vi "Angle overlay.vi"(8 "error in (no error)":errorcluster, 10 "Overlay details in":T2={"Text factor"=0, "Xoffset"=0, "Arc size"=0.0, "Result"=0.0, "Line width"=0, "Measurment Name"="", "Angle"={"Point 1"={"X"=0.0, "Y"=0.0}, "Point 2"={"X"=0.0, "Y"=0.0}, "vertex"={"X"=0.0, "Y"=0.0}, "Point 1a"={"X"=0.0, "Y"=0.0}, "Point 2a"={"X"=0.0, "Y"=0.0}, "line1Point1"={"X"=0.0, "Y"=0.0}, "line1Point2"={"X"=0.0, "Y"=0.0}, "line2Point1"={"X"=0.0, "Y"=0.0}, "line2Point2"={"X"=0.0, "Y"=0.0}, "Angle type"="theta"}, "Maintain Width?"=FALSE, "Size factor"=0, "Colour"=0, "Mouse release point"={"X"=0.0, "Y"=0.0}, "Small FOV?"=FALSE, "Fixed FOV parameters"={"Inspection mode"=FALSE, "Overlay coordinates"=[], "Config coordinates"=[]}}, 11 "Image in":T1) -> (0 "error out":errorcluster, 1 "Overlay Coordinates out":cluster{"X":sgl, "Y":sgl}[](array[cluster]), 2 "Text origin":cluster{"X":sgl, "Y":sgl}, 3 "Image out":T1)   [LabVIEW 2019]
uses:
  <vilib>/vision/Image Controls.llb/IMAQ Image.ctl
  Controls/Angle details.ctl
  <vilib>/vision/NI_Vision_Development_Module.lvlib
panel:
  out "Error out":errorcluster
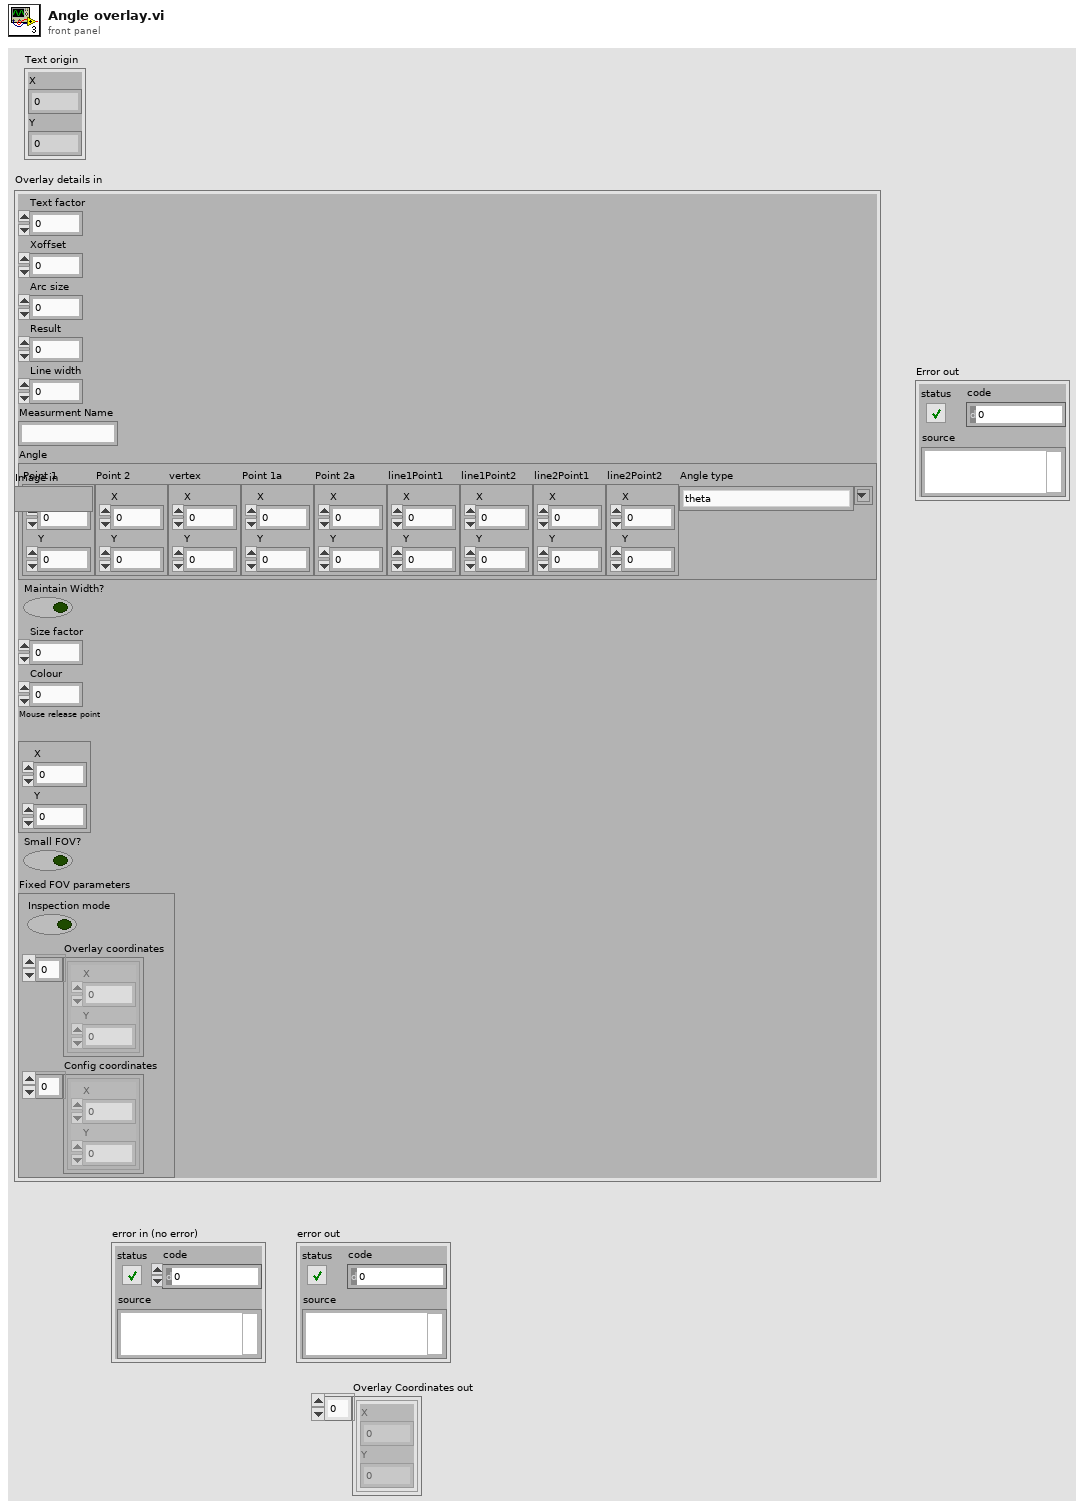
[diagram p1: front panel]
types:
  T1 = typedef "IMAQ Image.ctl" = refnum<image>
  T2 = typedef "Angle details.ctl" = cluster{"Text factor":u8, "Xoffset":i32, "Arc size":dbl, "Result":sgl, "Line width":i32, "Measurment Name":string, "Angle":cluster{"Point 1":cluster{"X":sgl, "Y":sgl}, "Point 2":cluster{"X":sgl, "Y":sgl}, "vertex":cluster{"X":sgl, "Y":sgl}, "Point 1a":cluster{"X":sgl, "Y":sgl}, "Point 2a":cluster{"X":sgl, "Y":sgl}, "line1Point1":cluster{"X":sgl, "Y":sgl}, "line1Point2":cluster{"X":sgl, "Y":sgl}, "line2Point1":cluster{"X":sgl, "Y":sgl}, "line2Point2":cluster{"X":sgl, "Y":sgl}, "Angle type":string}, "Maintain Width?":bool, "Size factor":u32, "Colour":u32, "Mouse release point":cluster{"X":sgl, "Y":sgl}, "Small FOV?":bool, "Fixed FOV parameters":cluster{"Inspection mode":bool, "Overlay coordinates":cluster{"X":sgl, "Y":sgl}[], "Config coordinates":cluster{"X":sgl, "Y":sgl}[]}}
  T3 = cluster{"Point 1":cluster{"X":sgl, "Y":sgl}, "Point 2":cluster{"X":sgl, "Y":sgl}}
  T4 = cluster{"Desired Font (Application)":enum16{"User-specified Font", "Application Font", "System Font", "Dialog Font"}, "[User-specified Font]":cluster{"Font Name":string, "Size":i16, "Strikeout?":bool, "Italic?":bool, "Underline?":bool, "Outline?":bool, "Shadow?":bool, "Bold?":bool, "Rotation Angle":dbl}, "Horizontal Alignment":i16, "Vertical Alignment":i16}
  T5 = cluster{"Point 1":cluster{"X":sgl, "Y":sgl}, "Point 2":cluster{"X":sgl, "Y":sgl}, "vertex":cluster{"X":sgl, "Y":sgl}, "Point 1a":cluster{"X":sgl, "Y":sgl}, "Point 2a":cluster{"X":sgl, "Y":sgl}, "line1Point1":cluster{"X":sgl, "Y":sgl}, "line1Point2":cluster{"X":sgl, "Y":sgl}, "line2Point1":cluster{"X":sgl, "Y":sgl}, "line2Point2":cluster{"X":sgl, "Y":sgl}, "Angle type":string}
  T6 = cluster{"Inspection mode":bool, "Overlay coordinates":cluster{"X":sgl, "Y":sgl}[], "Config coordinates":cluster{"X":sgl, "Y":sgl}[]}
  T7 = typedef "IMAQ Line" = cluster{"Start X":i32, "Start Y":i32, "End X":i32, "End Y":i32}
  T8 = cluster{"Left":i32, "Top":i32, "Right":i32, "Bottom":i32}
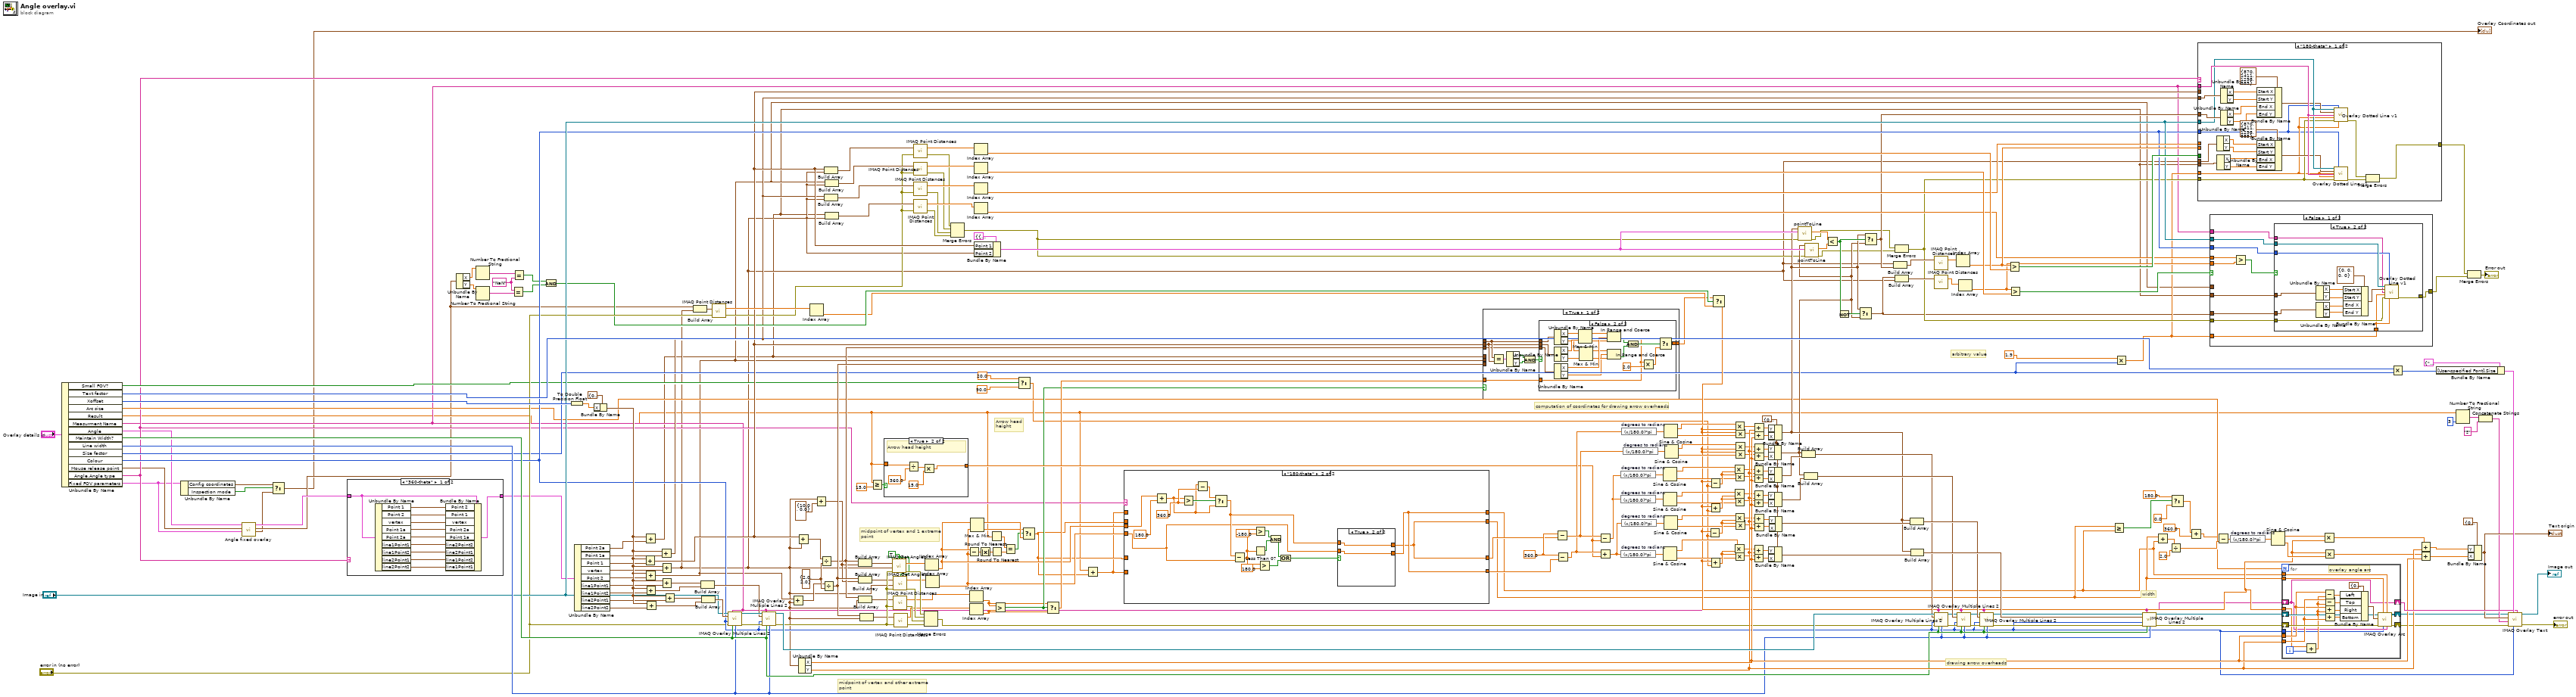
[diagram p0: block diagram]
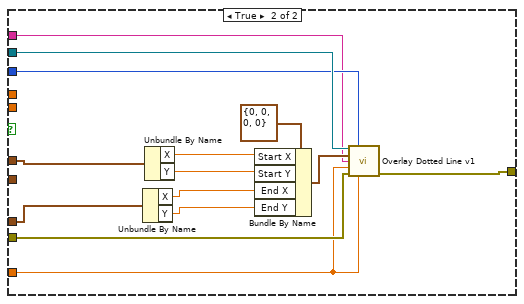
[diagram p3: hidden frame]
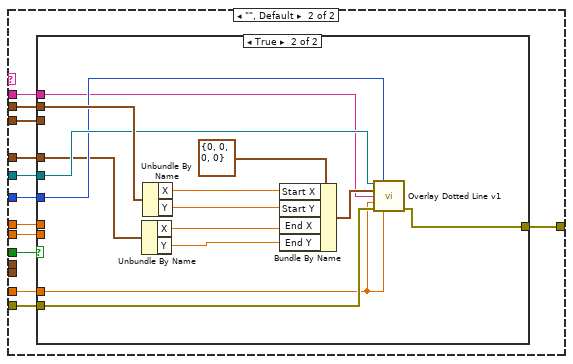
[diagram p4: hidden frame]
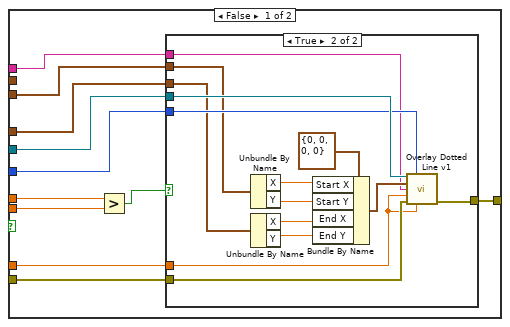
[diagram p5: hidden frame]
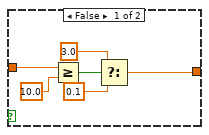
[diagram p10: hidden frame]
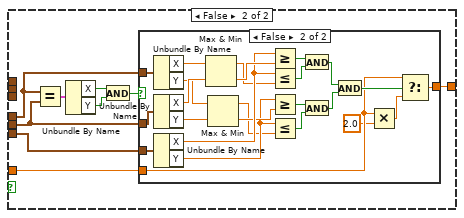
[diagram p12: hidden frame]
diagram:
  w48 = "NaN" ("x")
  w216 = 360.0 ("x")
  w198 = cluster{"X":sgl, "Y":sgl} {"X"=0.0, "Y"=0.0} ("y")
  w136 = cluster{"X":sgl, "Y":sgl} {"X"=2.0, "Y"=2.0} ("y")
  w110 = TRUE ("Use Vertex (No)")
  # "arbitrary value"
  # "Arrow head\nheight"
  # "midpoint of vertex and other extreme\npoint"
  # "midpoint of vertex and 1 extreme\npoint"
  # "drawing arrow overheads"
  # "computation of coordinates for drawing arrow overheads"
  # "width"
  n1 = Unbundle By Name("Overlay details in") -> ("Small FOV?"=w37:bool, "Text factor"=w104:u8, "Xoffset"=w103:i32, "Arc size"=w38:dbl, "Result"=w18:sgl, "Measurment Name"=w22:string, "Angle"=w9:T5, "Maintain Width?"=w102:bool, "Line width"=w101:i32, "Size factor"=w41:u32, "Colour"=w79:u32, "Mouse release point"=w7:cluster{"X":sgl, "Y":sgl}, "Angle.Angle type"=w23:string, "Fixed FOV parameters"=w5:T6)
  n2 = Unbundle By Name(w5) -> ("Config coordinates"=w3:cluster{"X":sgl, "Y":sgl}[], "Inspection mode"=w2:bool)
  n3 = call "Angle fixed overlay.vi"("Fixed FOV parameters"=w5, "Mouse release point"=w7, "Angle"=w9) -> ("Overlay Coordinates"=w4:cluster{"X":sgl, "Y":sgl}[], "Mouse release point out"=w6:cluster{"X":sgl, "Y":sgl}, "Angle parameters out"=w8:T5)  [unwired: 6 in]
  n4 = Select(t=w3, s=w2, f=w4) -> (s? t:f=→"Overlay Coordinates out":cluster{"X":sgl, "Y":sgl}[])
  n5 = case shown="\"360-theta\"" w23 {
    tunnel: w8 -> [w266 w267]
    tunnel: [w265 w267] -> w31
    frame "360-theta" {
      n6 = Unbundle By Name(w266) -> ("Point 1"=w264:cluster{"X":sgl, "Y":sgl}, "Point 2"=w263:cluster{"X":sgl, "Y":sgl}, "vertex"=w262:cluster{"X":sgl, "Y":sgl}, "Point 1a"=w261:cluster{"X":sgl, "Y":sgl}, "Point 2a"=w260:cluster{"X":sgl, "Y":sgl}, "line1Point1"=w259:cluster{"X":sgl, "Y":sgl}, "line1Point2"=w258:cluster{"X":sgl, "Y":sgl}, "line2Point1"=w257:cluster{"X":sgl, "Y":sgl}, "line2Point2"=w256:cluster{"X":sgl, "Y":sgl})
      n7 = Bundle By Name(cluster=w266, "Point 2"=w264, "Point 1"=w263, "vertex"=w262, "Point 2a"=w261, "Point 1a"=w260, "line2Point2"=w259, "line2Point1"=w258, "line1Point2"=w257, "line1Point1"=w256) -> (w265:T5)
    }
    frame "theta", Default {
    }
  }
  n8 = Unbundle By Name(w6) -> ("X"=w52:sgl, "Y"=w51:sgl)
  n9 = Number To Fractional String(number=w52) -> (F-format string=w50:string)  [unwired: 3 in]
  n10 = Number To Fractional String(number=w51) -> (F-format string=w49:string)  [unwired: 3 in]
  n11 = Equal?(x=w48, y=w49) -> (x = y?=w46:bool)
  n12 = Equal?(x=w50, y=w48) -> (x = y?=w47:bool)
  n13 = And(x=w47, y=w46) -> (x .and. y?=w45:bool)
  n14 = To Double Precision Float(number=w103) -> (double precision float=w234:dbl)
  n15 = Unbundle By Name(w31) -> ("Point 2a"=w235:cluster{"X":sgl, "Y":sgl}, "Point 1a"=w236:cluster{"X":sgl, "Y":sgl}, "Point 1"=w237:cluster{"X":sgl, "Y":sgl}, "vertex"=w33:cluster{"X":sgl, "Y":sgl}, "Point 2"=w238:cluster{"X":sgl, "Y":sgl}, "line1Point1"=w239:cluster{"X":sgl, "Y":sgl}, "line1Point2"=w241:cluster{"X":sgl, "Y":sgl}, "line2Point1"=w243:cluster{"X":sgl, "Y":sgl}, "line2Point2"=w246:cluster{"X":sgl, "Y":sgl})
  n16 = Bundle By Name(cluster=cluster{"X":sgl, "Y":sgl} {"X"=0.0, "Y"=0.0} ("Angle.Point 2a"), "X"=w234) -> (w245:cluster{"X":sgl, "Y":sgl})
  n17 = Add(x=w245, y=w237) -> (x+y=w75:cluster{"X":sgl, "Y":sgl})
  n18 = Add(x=w245, y=w235) -> (x+y=w19:cluster{"X":sgl, "Y":sgl})
  n19 = Add(x=w245, y=w238) -> (x+y=w21:cluster{"X":sgl, "Y":sgl})
  n20 = Add(x=w245, y=w241) -> (x+y=w242:cluster{"X":sgl, "Y":sgl})
  n21 = Add(x=w245, y=w246) -> (x+y=w247:cluster{"X":sgl, "Y":sgl})
  n22 = Add(x=w245, y=w236) -> (x+y=w24:cluster{"X":sgl, "Y":sgl})
  n23 = Add(x=w245, y=w33) -> (x+y=w20:cluster{"X":sgl, "Y":sgl})
  n24 = Add(x=w245, y=w239) -> (x+y=w240:cluster{"X":sgl, "Y":sgl})
  n25 = Add(x=w245, y=w243) -> (x+y=w244:cluster{"X":sgl, "Y":sgl})
  n26 = Build Array(w6, w20) -> (w78:cluster{"X":sgl, "Y":sgl}[])
  n27 = Build Array(w240, w242) -> (w232:cluster{"X":sgl, "Y":sgl}[])
  n28 = Build Array(w244, w247) -> (w248:cluster{"X":sgl, "Y":sgl}[])
  n29 = call "IMAQ Point Distances"("Points"=w78, "error in (no error)"="error in (no error)") -> ("Distances"=w77:sgl[], "error out"=w58:errorcluster)  [unwired: 3 in]
  n30 = call "IMAQ Overlay Multiple Lines 2"("Image"="Image in", "Group"=w22, "Line End Points"=w248, "Color"=w79, "error in (no error)"="error in (no error)", "Maintain Width?"=w102, "Width"=w101) -> ("Image Out"=w252:T1, "error out"=w251:errorcluster)  [unwired: 7 in]
  n31 = call "IMAQ Overlay Multiple Lines 2"("Image"=w252, "Group"=w22, "Line End Points"=w232, "Color"=w79, "error in (no error)"=w251, "Maintain Width?"=w102, "Width"=w101) -> ("Image Out"=w231:T1, "error out"=w230:errorcluster)  [unwired: 7 in]
  n32 = Add(x=w21, y=w20) -> (x+y=w135:cluster{"X":sgl, "Y":sgl})
  n33 = Add(x=w75, y=w20) -> (x+y=w219:cluster{"X":sgl, "Y":sgl})
  n34 = Unbundle By Name(w20) -> ("X"=w200:sgl, "Y"=w199:sgl)
  n35 = Index Array(array=w77) -> (element=w43:sgl)  [unwired: 1 in]
  n36 = Add(x=w20, y=cluster{"X":sgl, "Y":sgl} {"X"=10.0, "Y"=0.0}) -> (x+y=w109:cluster{"X":sgl, "Y":sgl})
  n37 = Divide(x=w219, y=w136) -> (x/y=w154:cluster{"X":sgl, "Y":sgl})
  n38 = Divide(x=w135, y=w136) -> (x/y=w155:cluster{"X":sgl, "Y":sgl})
  n39 = Build Array(w75, w20) -> (w100:cluster{"X":sgl, "Y":sgl}[])
  n40 = Build Array(w24, w20) -> (w98:cluster{"X":sgl, "Y":sgl}[])
  n41 = Build Array(w21, w20) -> (w99:cluster{"X":sgl, "Y":sgl}[])
  n42 = Build Array(w19, w20) -> (w97:cluster{"X":sgl, "Y":sgl}[])
  n43 = Build Array(w154, w109) -> (w106:cluster{"X":sgl, "Y":sgl}[])
  n44 = Build Array(w155, w109) -> (w107:cluster{"X":sgl, "Y":sgl}[])
  n45 = Build Array(w154, w20) -> (w113:cluster{"X":sgl, "Y":sgl}[])
  n46 = Build Array(w155, w20) -> (w114:cluster{"X":sgl, "Y":sgl}[])
  n47 = Greater Or Equal?(x=w18, y=sgl 15.0) -> (x >= y?=w176:bool)
  n48 = case shown="True" w176 {
    tunnel: w18 -> [w273 w278]
    tunnel: [w268 w274] -> w177
    frame False {
      n49 = Greater Or Equal?(x=w273, y=sgl 10.0) -> (x >= y?=w271:bool)
      n50 = Select(t=3.0, s=w271, f=0.1) -> (s? t:f=w268:dbl)
    }
    frame True {
      # "Arrow head height"
      n51 = Divide(x=w278, y=sgl 360.0) -> (x/y=w276:sgl)
      n52 = Multiply(x=w276, y=sgl 15.0) -> (x*y=w274:sgl)
    }
  }
  n53 = call "IMAQ Get Angles"("error in (no error)"=w230, "Vertex"=w20, "Points"=w106, "Use Vertex (No)"=w110) -> ("error out"=w141:errorcluster, "Angles (deg)"=w111:sgl[])  [unwired: 1 in, 1 out]
  n54 = call "IMAQ Get Angles"("error in (no error)"=w230, "Vertex"=w20, "Points"=w107, "Use Vertex (No)"=w110) -> ("error out"=w140:errorcluster, "Angles (deg)"=w112:sgl[])  [unwired: 1 in, 1 out]
  n55 = call "IMAQ Point Distances"("Points"=w113, "error in (no error)"=w230) -> ("Distances"=w115:sgl[], "error out"=w139:errorcluster)  [unwired: 3 in]
  n56 = call "IMAQ Point Distances"("Points"=w114, "error in (no error)"=w230) -> ("Distances"=w116:sgl[], "error out"=w138:errorcluster)  [unwired: 3 in]
  n57 = call "IMAQ Point Distances"("Points"=w100, "error in (no error)"=w58) -> ("Distances"=w94:sgl[], "error out"=w54:errorcluster)  [unwired: 3 in]
  n58 = call "IMAQ Point Distances"("Points"=w98, "error in (no error)"=w58) -> ("Distances"=w92:sgl[], "error out"=w56:errorcluster)  [unwired: 3 in]
  n59 = call "IMAQ Point Distances"("Points"=w99, "error in (no error)"=w58) -> ("Distances"=w93:sgl[], "error out"=w55:errorcluster)  [unwired: 3 in]
  n60 = call "IMAQ Point Distances"("Points"=w97, "error in (no error)"=w58) -> ("Distances"=w91:sgl[], "error out"=w57:errorcluster)  [unwired: 3 in]
  n61 = Merge Errors(w141, w140, w139, w138) -> (w66:errorcluster)
  n62 = Index Array(array=w111) -> (element=w30:sgl)  [unwired: 1 in]
  n63 = Index Array(array=w112) -> (element=w29:sgl)  [unwired: 1 in]
  n64 = Merge Errors(w54, w55, w56, w57) -> (w53:errorcluster)
  n65 = Subtract(x=w30, y=w29) -> (x-y=w223:sgl)
  n66 = Index Array(array=w115) -> (element=w117:sgl)  [unwired: 1 in]
  n67 = Index Array(array=w116) -> (element=w118:sgl)  [unwired: 1 in]
  n68 = Max & Min(x=w30, y=w29) -> (max(x,y)=w226:sgl, min(x,y)=w225:sgl)
  n69 = Index Array(array=w94) -> (element=w89:sgl)  [unwired: 1 in]
  n70 = Index Array(array=w93) -> (element=w87:sgl)  [unwired: 1 in]
  n71 = Index Array(array=w92) -> (element=w84:sgl)  [unwired: 1 in]
  n72 = Index Array(array=w91) -> (element=w82:sgl)  [unwired: 1 in]
  n73 = Bundle By Name(cluster=T3 {"Point 1"={"X"=0.0, "Y"=0.0}, "Point 2"={"X"=0.0, "Y"=0.0}} ("Line"), "Point 1"=w75, "Point 2"=w20) -> (w74:T3)
  n74 = Absolute Value(x=w223) -> (abs(x)=w228:sgl)
  n75 = Round To Nearest(number=w18) -> (nearest integer value=w229:sgl)
  n76 = Round To Nearest(number=w228) -> (nearest integer value=w227:sgl)
  n77 = Greater?(x=w117, y=w118) -> (0:w153:bool)
  n78 = Equal?(x=w229, y=w227) -> (x = y?=w224:bool)
  n79 = Select(t=sgl 20.0 ("y"), s=w37, f=sgl 90.0 ("y")) -> (s? t:f=w34:sgl)
  n80 = Select(t=w225, s=w224, f=w226) -> (s? t:f=w28:sgl)
  n81 = Select(t=w117, s=w153, f=w118) -> (s? t:f=w156:sgl)
  n82 = Add(x=w18, y=w28) -> (x+y=w26:sgl)
  n83 = case shown="\"180-theta\"" w23 {
    tunnel: w28 -> [w281 _]
    tunnel: w26 -> [w282 _]
    tunnel: w30 -> [_ w295]
    tunnel: w29 -> [_ w290]
    tunnel: [w282 w289] -> w11
    tunnel: [w281 w288] -> w12
    tunnel: w28 -> [w280 _]
    tunnel: [w280 w288] -> w27
    tunnel: [w279 w289] -> w25
    tunnel: w26 -> [w279 _]
    frame "", Default {
    }
    frame "180-theta" {
      w297 = sgl 360.0 ("y")
      n84 = Add(x=w295, y=sgl 180.0) -> (x+y=w296:sgl)
      n85 = Greater?(x=w296, y=w297) -> (0:w299:bool)
      n86 = Subtract(x=w296, y=w297) -> (x-y=w298:sgl)
      n87 = Select(t=w298, s=w299, f=w296) -> (s? t:f=w291:sgl)
      n88 = Subtract(x=w291, y=w290) -> (x-y=w287:sgl)
      n89 = Greater?(x=w287, y=sgl -180.0) -> (0:w285:bool)
      n90 = Less Than 0?(x=w287) -> (x < 0?=w284:bool)
      n91 = Greater?(x=w287, y=sgl 180.0) -> (0:w293:bool)
      n92 = And(x=w285, y=w284) -> (x .and. y?=w283:bool)
      n93 = Or(x=w283, y=w293) -> (x .or. y?=w292:bool)
      n94 = case shown="True" w292 {
        tunnel: w291 -> [w302 w303]
        tunnel: w290 -> [w301 w304]
        tunnel: [w302 w304] -> w289
        tunnel: [w301 w303] -> w288
        frame False {
        }
        frame True {
        }
      }
    }
  }
  n95 = case shown="True" w153 {
    tunnel: w75 -> [w310 _]
    tunnel: w24 -> [w311 _]
    tunnel: w21 -> [_ w339]
    tunnel: w19 -> [_ w340]
    tunnel: w154 -> [w305 _]
    tunnel: w155 -> [_ w341]
    tunnel: w156 -> [w312 w343]
    tunnel: [w313 w342] -> w42
    frame True {
      n96 = Equal?(x=w311, y=w310) -> (x = y?=w309:cluster{"X":bool, "Y":bool})
      n97 = Unbundle By Name(w309) -> ("X"=w308:bool, "Y"=w307:bool)
      n98 = And(x=w308, y=w307) -> (x .and. y?=w306:bool)
      n99 = case shown="False" w306 {
        tunnel: w305 -> [_ w334]
        tunnel: [w314 w326] -> w313
        tunnel: w312 -> [w314 w325]
        tunnel: w311 -> [_ w324]
        tunnel: w310 -> [_ w323]
        frame True {
        }
        frame False {
          n100 = Unbundle By Name(w324) -> ("X"=w333:sgl, "Y"=w331:sgl)
          n101 = Unbundle By Name(w323) -> ("X"=w332:sgl, "Y"=w330:sgl)
          n102 = Unbundle By Name(w334) -> ("X"=w321:sgl, "Y"=w316:sgl)
          n103 = Max & Min(x=w333, y=w332) -> (max(x,y)=w322:sgl, min(x,y)=w320:sgl)
          n104 = Max & Min(x=w331, y=w330) -> (max(x,y)=w318:sgl, min(x,y)=w317:sgl)
          n105 = In Range and Coerce(upper limit=w322, x=w321, lower limit=w320) -> (In Range?=w319:bool)  [unwired: 1 out]
          n106 = In Range and Coerce(upper limit=w318, x=w316, lower limit=w317) -> (In Range?=w315:bool)  [unwired: 1 out]
          n107 = And(x=w319, y=w315) -> (x .and. y?=w329:bool)
          n108 = Multiply(x=w325, y=sgl 2.0) -> (x*y=w328:sgl)
          n109 = Select(t=w325, s=w329, f=w328) -> (s? t:f=w326:sgl)
        }
      }
    }
    frame False {
      n110 = Equal?(x=w340, y=w339) -> (x = y?=w338:cluster{"X":bool, "Y":bool})
      n111 = Unbundle By Name(w338) -> ("X"=w337:bool, "Y"=w336:bool)
      n112 = And(x=w337, y=w336) -> (x .and. y?=w335:bool)
      n113 = case shown="False" w335 {
        tunnel: w343 -> [w344 w350]
        tunnel: [w344 w348] -> w342
        tunnel: w341 -> [_ w347]
        tunnel: w340 -> [_ w346]
        tunnel: w339 -> [_ w345]
        frame True {
        }
        frame False {
          n114 = Unbundle By Name(w346) -> ("X"=w368:sgl, "Y"=w366:sgl)
          n115 = Unbundle By Name(w345) -> ("X"=w367:sgl, "Y"=w365:sgl)
          n116 = Unbundle By Name(w347) -> ("X"=w363:sgl, "Y"=w356:sgl)
          n117 = Max & Min(x=w368, y=w367) -> (max(x,y)=w362:sgl, min(x,y)=w364:sgl)
          n118 = Max & Min(x=w366, y=w365) -> (max(x,y)=w355:sgl, min(x,y)=w357:sgl)
          n119 = Greater Or Equal?(x=w363, y=w364) -> (x >= y?=w361:bool)
          n120 = Less Or Equal?(x=w363, y=w362) -> (x <= y?=w360:bool)
          n121 = Greater Or Equal?(x=w356, y=w357) -> (x >= y?=w358:bool)
          n122 = Less Or Equal?(x=w356, y=w355) -> (x <= y?=w359:bool)
          n123 = And(x=w361, y=w360) -> (x .and. y?=w353:bool)
          n124 = And(x=w358, y=w359) -> (x .and. y?=w354:bool)
          n125 = And(x=w353, y=w354) -> (x .and. y?=w352:bool)
          n126 = Multiply(x=w350, y=sgl 2.0) -> (x*y=w351:sgl)
          n127 = Select(t=w350, s=w352, f=w351) -> (s? t:f=w348:sgl)
        }
      }
    }
  }
  n128 = Subtract(x=w216, y=w27) -> (x-y=w218:dbl)
  n129 = Subtract(x=w216, y=w25) -> (x-y=w217:dbl)
  n130 = Subtract(x=w218, y=w177) -> (x-y=w249:dbl)
  n131 = Add(x=w217, y=w177) -> (x+y=w215:dbl)
  n132 = expression code="(x/180.0)*pi" "degrees to radians"(w249) -> (w157:dbl)
  n133 = expression code="(x/180.0)*pi" "degrees to radians"(w249) -> (w181:dbl)
  n134 = expression code="(x/180.0)*pi" "degrees to radians"(w215) -> (w190:dbl)
  n135 = expression code="(x/180.0)*pi" "degrees to radians"(w217) -> (w143:dbl)
  n136 = expression code="(x/180.0)*pi" "degrees to radians"(w215) -> (w162:dbl)
  n137 = expression code="(x/180.0)*pi" "degrees to radians"(w218) -> (w144:dbl)
  n138 = Sine & Cosine(0:w157) -> (1:w158:dbl, 2:w159:dbl)
  n139 = Sine & Cosine(0:w181) -> (1:w182:dbl, 2:w183:dbl)
  n140 = Sine & Cosine(0:w190) -> (1:w191:dbl, 2:w192:dbl)
  n141 = Sine & Cosine(0:w143) -> (1:w145:dbl, 2:w146:dbl)
  n142 = Sine & Cosine(0:w162) -> (1:w163:dbl, 2:w164:dbl)
  n143 = Sine & Cosine(0:w144) -> (1:w147:dbl, 2:w148:dbl)
  n144 = Select(t=w42, s=w45, f=w43) -> (s? t:f=w44:sgl)
  n145 = Subtract(x=w44, y=w34) -> (x-y=w189:sgl)
  n146 = Subtract(x=w44, y=w34) -> (x-y=w180:sgl)
  n147 = Add(x=w44, y=w34) -> (x+y=w188:sgl)
  n148 = Add(x=w44, y=w34) -> (x+y=w197:sgl)
  n149 = Multiply(x=w158, y=w180) -> (x*y=w160:dbl)
  n150 = Multiply(x=w182, y=w188) -> (x*y=w184:dbl)
  n151 = Multiply(x=w191, y=w197) -> (x*y=w193:dbl)
  n152 = Multiply(x=w145, y=w44) -> (x*y=w149:dbl)
  n153 = Multiply(x=w180, y=w159) -> (x*y=w161:dbl)
  n154 = Multiply(x=w188, y=w183) -> (x*y=w185:dbl)
  n155 = Multiply(x=w163, y=w189) -> (x*y=w165:dbl)
  n156 = Multiply(x=w197, y=w192) -> (x*y=w194:dbl)
  n157 = Multiply(x=w44, y=w146) -> (x*y=w150:dbl)
  n158 = Multiply(x=w147, y=w44) -> (x*y=w151:dbl)
  n159 = Multiply(x=w44, y=w148) -> (x*y=w152:dbl)
  n160 = Multiply(x=w189, y=w164) -> (x*y=w166:dbl)
  n161 = Add(x=w160, y=w199) -> (x+y=w171:dbl)
  n162 = Add(x=w161, y=w200) -> (x+y=w172:dbl)
  n163 = Add(x=w184, y=w199) -> (x+y=w186:dbl)
  n164 = Add(x=w185, y=w200) -> (x+y=w187:dbl)
  n165 = Add(x=w193, y=w199) -> (x+y=w195:dbl)
  n166 = Add(x=w194, y=w200) -> (x+y=w196:dbl)
  n167 = Add(x=w149, y=w199) -> (x+y=w167:dbl)
  n168 = Add(x=w150, y=w200) -> (x+y=w168:dbl)
  n169 = Add(x=w151, y=w199) -> (x+y=w169:dbl)
  n170 = Add(x=w152, y=w200) -> (x+y=w170:dbl)
  n171 = Add(x=w165, y=w199) -> (x+y=w173:dbl)
  n172 = Add(x=w166, y=w200) -> (x+y=w174:dbl)
  n173 = Bundle By Name(cluster=w198, "Y"=w169, "X"=w170) -> (w68:cluster{"X":sgl, "Y":sgl})
  n174 = Bundle By Name(cluster=w198, "Y"=w167, "X"=w168) -> (w69:cluster{"X":sgl, "Y":sgl})
  n175 = Bundle By Name(cluster=w198, "Y"=w171, "X"=w172) -> (w201:cluster{"X":sgl, "Y":sgl})
  n176 = Bundle By Name(cluster=w198, "Y"=w186, "X"=w187) -> (w202:cluster{"X":sgl, "Y":sgl})
  n177 = Bundle By Name(cluster=w198, "Y"=w195, "X"=w196) -> (w204:cluster{"X":sgl, "Y":sgl})
  n178 = Bundle By Name(cluster=w198, "Y"=w173, "X"=w174) -> (w203:cluster{"X":sgl, "Y":sgl})
  n179 = call "pointToLine.vi"("error in (no error)"=w53, "Line"=w74, "Point"=w69) -> ("error out"=w64:errorcluster, "distance"=w73:dbl)  [unwired: 6 in, 1 out]
  n180 = Build Array(w68, w201) -> (w211:cluster{"X":sgl, "Y":sgl}[])
  n181 = Build Array(w68, w202) -> (w212:cluster{"X":sgl, "Y":sgl}[])
  n182 = call "pointToLine.vi"("error in (no error)"=w53, "Line"=w74, "Point"=w68) -> ("error out"=w65:errorcluster, "distance"=w72:dbl)  [unwired: 6 in, 1 out]
  n183 = Less?(x=w73, y=w72) -> (x < y?=w71:bool)
  n184 = Not(x=w71) -> (.not. x?=w70:bool)
  n185 = Select(t=w69, s=w70, f=w68) -> (s? t:f=w32:cluster{"X":sgl, "Y":sgl})
  n186 = Select(t=w69, s=w71, f=w68) -> (s? t:f=w67:cluster{"X":sgl, "Y":sgl})
  n187 = Build Array(w20, w67) -> (w96:cluster{"X":sgl, "Y":sgl}[])
  n188 = Build Array(w32, w20) -> (w95:cluster{"X":sgl, "Y":sgl}[])
  n189 = Merge Errors(w64, w65) -> (w63:errorcluster)
  n190 = Build Array(w69, w203) -> (w213:cluster{"X":sgl, "Y":sgl}[])
  n191 = Build Array(w69, w204) -> (w214:cluster{"X":sgl, "Y":sgl}[])
  n192 = call "IMAQ Point Distances"("Points"=w96) -> ("Distances"=w90:sgl[])  [unwired: 4 in, 1 out]
  n193 = call "IMAQ Overlay Multiple Lines 2"("Image"=w231, "Group"=w22, "Line End Points"=w211, "Color"=w79, "error in (no error)"=w66, "Maintain Width?"=w102, "Width"=w101) -> ("Image Out"=w179:T1, "error out"=w178:errorcluster)  [unwired: 7 in]
  n194 = call "IMAQ Point Distances"("Points"=w95) -> ("Distances"=w88:sgl[])  [unwired: 4 in, 1 out]
  n195 = Index Array(array=w90) -> (element=w83:sgl)  [unwired: 1 in]
  n196 = call "IMAQ Overlay Multiple Lines 2"("Image"=w179, "Group"=w22, "Line End Points"=w212, "Color"=w79, "error in (no error)"=w178, "Maintain Width?"=w102, "Width"=w101) -> ("Image Out"=w206:T1, "error out"=w205:errorcluster)  [unwired: 7 in]
  n197 = Index Array(array=w88) -> (element=w81:sgl)  [unwired: 1 in]
  n198 = call "IMAQ Overlay Multiple Lines 2"("Image"=w206, "Group"=w22, "Line End Points"=w213, "Color"=w79, "error in (no error)"=w205, "Maintain Width?"=w102, "Width"=w101) -> ("Image Out"=w209:T1, "error out"=w207:errorcluster)  [unwired: 7 in]
  n199 = Greater?(x=w83, y=w89) -> (0:w86:bool)
  n200 = Greater?(x=w81, y=w87) -> (0:w85:bool)
  n201 = Greater Or Equal?(x=w12, y=w11) -> (x >= y?=w10:bool)
  n202 = Multiply(x=1.9, y=w41) -> (x*y=w40:dbl)
  n203 = call "IMAQ Overlay Multiple Lines 2"("Image"=w209, "Group"=w22, "Line End Points"=w214, "Color"=w79, "error in (no error)"=w207, "Maintain Width?"=w102, "Width"=w101) -> ("Image Out"=w210:T1, "error out"=w208:errorcluster)  [unwired: 7 in]
  n204 = Add(x=w12, y=w11) -> (x+y=w124:sgl)
  n205 = Divide(x=w124, y=2.0) -> (x/y=w221:dbl)
  n206 = Select(t=180.0, s=w10, f=0.0) -> (s? t:f=w13:dbl)
  n207 = Add(x=w13, y=360.0 ("x")) -> (x+y=w17:dbl)
  n208 = case shown="\"180-theta\"" w23 {
    tunnel: w86 -> [_ w404]
    tunnel: w84 -> [_ w403]
    tunnel: w83 -> [_ w402]
    tunnel: "Image in" -> [w377 w401]
    tunnel: w79 -> [w369 w400]
    tunnel: w75 -> [_ w399]
    tunnel: w67 -> [w391 w398]
    tunnel: w63 -> [w374 w397]
    tunnel: [w371 w396] -> w61
    tunnel: w40 -> [w373 w395]
    tunnel: w22 -> [w378 w394]
    tunnel: w24 -> [w386 w393]
    tunnel: w19 -> [w385 _]
    tunnel: w20 -> [w384 _]
    frame "180-theta" {
      n209 = Unbundle By Name(w384) -> ("X"=w382:sgl, "Y"=w381:sgl)
      n210 = Unbundle By Name(w385) -> ("X"=w380:sgl, "Y"=w379:sgl)
      n211 = Unbundle By Name(w386) -> ("X"=w390:sgl, "Y"=w389:sgl)
      n212 = Unbundle By Name(w391) -> ("X"=w388:sgl, "Y"=w387:sgl)
      n213 = Bundle By Name(cluster=T7 {"Start X"=870, "Start Y"=1411, "End X"=1298, "End Y"=885} ("Line"), "Start X"=w390, "Start Y"=w389, "End X"=w388, "End Y"=w387) -> (w376:T7)
      n214 = Bundle By Name(cluster=T7 {"Start X"=870, "Start Y"=1411, "End X"=1298, "End Y"=885} ("Line"), "Start X"=w382, "Start Y"=w381, "End X"=w380, "End Y"=w379) -> (w375:T7)
      n215 = call "Overlay Dotted Line v1.vi"("Imae in"=w377, "Color"=w369, "Line"=w376, "Measurement Name"=w378, "alternative factor"=w373, "error in (no error)"=w374, "Point Diameter (5)"=w373) -> ("error out"=w370:errorcluster)  [unwired: 7 in, 1 out]
      n216 = call "Overlay Dotted Line v1.vi"("Imae in"=w377, "Color"=w369, "Line"=w375, "Measurement Name"=w378, "alternative factor"=w373, "error in (no error)"=w374, "Point Diameter (5)"=w373) -> ("error out"=w372:errorcluster)  [unwired: 7 in, 1 out]
      n217 = Merge Errors(w370, w372) -> (w371:errorcluster)
    }
    frame "", Default {
      n218 = case shown="True" w404 {
        tunnel: w403 -> [w415 _]
        tunnel: w402 -> [w414 _]
        tunnel: w401 -> [w412 w437]
        tunnel: w400 -> [w411 w436]
        tunnel: w399 -> [_ w444]
        tunnel: w393 -> [w409 _]
        tunnel: w398 -> [w410 w435]
        tunnel: w397 -> [w408 w434]
        tunnel: [w407 w433] -> w396
        tunnel: w395 -> [w406 w431]
        tunnel: w394 -> [w405 w432]
        frame False {
          n219 = Greater?(x=w415, y=w414) -> (0:w413:bool)
          n220 = case shown="True" w413 {
            tunnel: w412 -> [_ w428]
            tunnel: w411 -> [_ w427]
            tunnel: w410 -> [_ w425]
            tunnel: w409 -> [_ w426]
            tunnel: w408 -> [w416 w420]
            tunnel: [w416 w419] -> w407
            tunnel: w406 -> [_ w418]
            tunnel: w405 -> [_ w417]
            frame False {
            }
            frame True {
              n221 = Unbundle By Name(w426) -> ("X"=w424:sgl, "Y"=w423:sgl)
              n222 = Unbundle By Name(w425) -> ("X"=w422:sgl, "Y"=w421:sgl)
              n223 = Bundle By Name(cluster=T7 {"Start X"=0, "Start Y"=0, "End X"=0, "End Y"=0} ("Line"), "Start X"=w424, "Start Y"=w423, "End X"=w422, "End Y"=w421) -> (w429:T7)
              n224 = call "Overlay Dotted Line v1.vi"("Imae in"=w428, "Color"=w427, "Line"=w429, "Measurement Name"=w417, "alternative factor"=w418, "error in (no error)"=w420, "Point Diameter (5)"=w418) -> ("error out"=w419:errorcluster)  [unwired: 7 in, 1 out]
            }
          }
        }
        frame True {
          n225 = Unbundle By Name(w435) -> ("X"=w441:sgl, "Y"=w440:sgl)
          n226 = Unbundle By Name(w444) -> ("X"=w443:sgl, "Y"=w442:sgl)
          n227 = Bundle By Name(cluster=T7 {"Start X"=0, "Start Y"=0, "End X"=0, "End Y"=0} ("Line"), "Start X"=w443, "Start Y"=w442, "End X"=w441, "End Y"=w440) -> (w438:T7)
          n228 = call "Overlay Dotted Line v1.vi"("Imae in"=w437, "Color"=w436, "Line"=w438, "Measurement Name"=w432, "alternative factor"=w431, "error in (no error)"=w434, "Point Diameter (5)"=w431) -> ("error out"=w433:errorcluster)  [unwired: 7 in, 1 out]
        }
      }
    }
  }
  n229 = case shown="False" w85 {
    tunnel: w82 -> [w455 _]
    tunnel: w81 -> [w454 _]
    tunnel: "Image in" -> [w452 w482]
    tunnel: w79 -> [w451 w481]
    tunnel: w21 -> [_ w480]
    tunnel: w19 -> [w449 _]
    tunnel: w32 -> [w450 w479]
    tunnel: w63 -> [w448 w474]
    tunnel: [w447 w473] -> w62
    tunnel: w40 -> [w446 w471]
    tunnel: w22 -> [w445 w472]
    frame False {
      n230 = Greater?(x=w455, y=w454) -> (0:w453:bool)
      n231 = case shown="True" w453 {
        tunnel: w452 -> [_ w462]
        tunnel: w451 -> [_ w461]
        tunnel: w450 -> [_ w463]
        tunnel: w449 -> [_ w464]
        tunnel: w448 -> [w456 w460]
        tunnel: [w456 w459] -> w447
        tunnel: w446 -> [_ w458]
        tunnel: w445 -> [_ w457]
        frame False {
        }
        frame True {
          n232 = Unbundle By Name(w464) -> ("X"=w467:sgl, "Y"=w468:sgl)
          n233 = Unbundle By Name(w463) -> ("X"=w469:sgl, "Y"=w470:sgl)
          n234 = Bundle By Name(cluster=T7 {"Start X"=0, "Start Y"=0, "End X"=0, "End Y"=0} ("Line"), "Start X"=w467, "Start Y"=w468, "End X"=w469, "End Y"=w470) -> (w466:T7)
          n235 = call "Overlay Dotted Line v1.vi"("Imae in"=w462, "Color"=w461, "Line"=w466, "Measurement Name"=w457, "alternative factor"=w458, "error in (no error)"=w460, "Point Diameter (5)"=w458) -> ("error out"=w459:errorcluster)  [unwired: 7 in, 1 out]
        }
      }
    }
    frame True {
      n236 = Unbundle By Name(w479) -> ("X"=w476:sgl, "Y"=w475:sgl)
      n237 = Unbundle By Name(w480) -> ("X"=w478:sgl, "Y"=w477:sgl)
      n238 = Bundle By Name(cluster=T7 {"Start X"=0, "Start Y"=0, "End X"=0, "End Y"=0} ("Line"), "Start X"=w478, "Start Y"=w477, "End X"=w476, "End Y"=w475) -> (w483:T7)
      n239 = call "Overlay Dotted Line v1.vi"("Imae in"=w482, "Color"=w481, "Line"=w483, "Measurement Name"=w472, "alternative factor"=w471, "error in (no error)"=w474, "Point Diameter (5)"=w471) -> ("error out"=w473:errorcluster)  [unwired: 7 in, 1 out]
    }
  }
  n240 = Subtract(x=w17, y=w221) -> (x-y=w222:dbl)
  n241 = expression code="(x/180.0)*pi" "degrees to radians"(w222) -> (w126:dbl)
  n242 = Sine & Cosine(0:w126) -> (1:w127:dbl, 2:w128:dbl)
  n243 = for {
    N: w38 -> [_]
    tunnel: w11 -> [w493]
    tunnel: w12 -> [w492]
    tunnel: w199 -> [w491]
    tunnel: w200 -> [w490]
    tunnel: w44 -> [w488]
    shift-right: [w497] -> w119
    shift-left: w210 -> [w495]
    shift-right: [w496] -> w134
    shift-left: w208 -> [w494]
    tunnel: w79 -> [w485]
    shift-right: [w486] -> w250
    shift-left: w22 -> [w486]
    i -> [w489]
    # "overlay angle arc"
    n244 = Add(x=w488, y=w489) -> (x+y=w487:sgl)
    n245 = Subtract(x=w490, y=w487) -> (x-y=w503:sgl)
    n246 = Subtract(x=w491, y=w487) -> (x-y=w502:sgl)
    n247 = Add(x=w490, y=w487) -> (x+y=w501:sgl)
    n248 = Add(x=w487, y=w491) -> (x+y=w500:sgl)
    n249 = Bundle By Name(cluster=T8 {"Left"=0, "Top"=0, "Right"=0, "Bottom"=0} ("Bounding Rectangle"), "Left"=w503, "Top"=w502, "Right"=w501, "Bottom"=w500) -> (w498:T8)
    n250 = call "IMAQ Overlay Arc"("Group"=w486, "End Angle (degrees)"=w493, "Color"=w485, "Start Angle (degrees)"=w492, "error in (no error)"=w494, "Bounding Rectangle"=w498, "Image"=w495) -> ("error out"=w496:errorcluster, "Image Out"=w497:T1)  [unwired: 3 in]
  }
  n251 = Multiply(x=w127, y=w44) -> (x*y=w133:dbl)
  n252 = Multiply(x=w44, y=w128) -> (x*y=w132:dbl)
  n253 = Multiply(x=w104, y=w41) -> (x*y=w255:u32)
  n254 = Add(x=w133, y=w199) -> (x+y=w142:dbl)
  n255 = Add(x=w132, y=w200) -> (x+y=w130:dbl)
  n256 = Bundle By Name(cluster=T4 {"Desired Font (Application)"=enum."User-specified Font", "[User-specified Font]"={"Font Name"="", "Size"=40, "Strikeout?"=FALSE, "Italic?"=FALSE, "Underline?"=FALSE, "Outline?"=FALSE, "Shadow?"=FALSE, "Bold?"=TRUE, "Rotation Angle"=0.0}, "Horizontal Alignment"=1, "Vertical Alignment"=2} ("Font, Size & Style"), "[User-specified Font].Size"=w255) -> (w254:T4)
  n257 = Number To Fractional String(number=w18, precision (6)=i16 3) -> (F-format string=w122:string)  [unwired: 2 in]
  n258 = Merge Errors(w61, w62) -> (→"Error out":errorcluster)
  n259 = Bundle By Name(cluster=cluster{"X":sgl, "Y":sgl} {"X"=0.0, "Y"=0.0} ("y"), "Y"=w142, "X"=w130) -> (w131:cluster{"X":sgl, "Y":sgl})
  "Text origin" <- w131
  n260 = Concatenate Strings(w122, "º" ("string")) -> (w123:string)
  n261 = call "IMAQ Overlay Text"("Group"=w250, "Text Color (black)"=w79, "Font, Size & Style"=w254, "error in (no error)"=w134, "String"=w123, "Origin"=w131, "Image"=w119) -> ("error out"=→"error out":errorcluster, "Image Out"=→"Image out":T1)  [unwired: 3 in]
